vi "temp_dir_generate.vi"(8 "error in (no error)":errorcluster, 11 "temp_dir_config":T1) -> (0 "error out":errorcluster, 3 "temp_dir":path)   [LabVIEW 2015, in "lv-post-installer.lvlib"]
uses:
  lv-post-installer.lvlib
  _controls/temp_dir_config.ctl
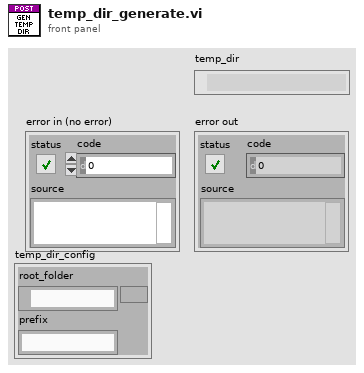
[diagram p1: front panel]
types:
  T1 = typedef "lv-post-installer.lvlib/temp_dir_config.ctl" = cluster{"root_folder":path, "prefix":string}
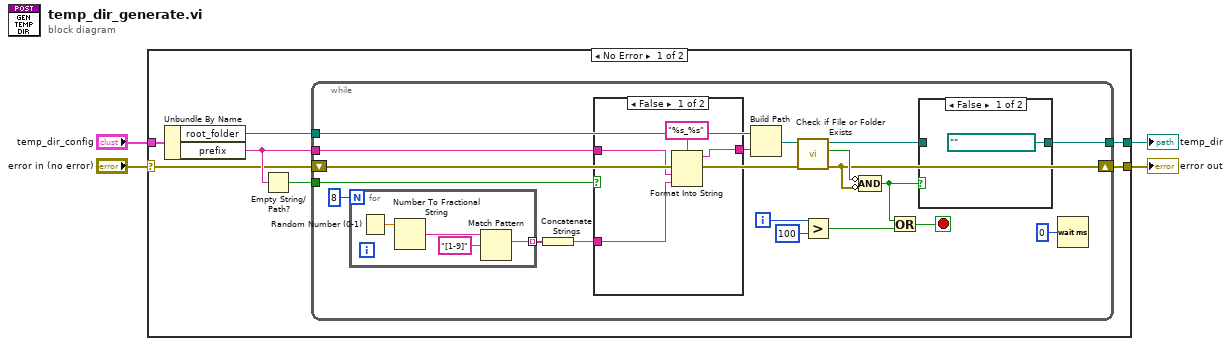
[diagram p0: block diagram]
diagram:
  n1 = case shown="No Error" "error in (no error)" {
    selector: "error in (no error)" -> [w5 w42]
    tunnel: [w8 _] -> w3
    tunnel: [w7 w42] -> w2
    tunnel: "temp_dir_config" -> [w6 _]
    frame No Error {
      n2 = Unbundle By Name(w6) -> ("root_folder"=w11:path, "prefix"=w10:string)
      n3 = Empty String/Path?(string/path=w10) -> (empty?=w9:bool)
      n4 = while {
        tunnel: w10 -> [w27]
        tunnel: w11 -> [w28]
        tunnel: w9 -> [w26]
        shift-right: [w21] -> w7
        shift-left: w5 -> [w12]
        tunnel: [w14] -> w8
        i -> [w19]
        stop <- w20 stop-if-true
        n5 = for {
          N: 8 -> [_]
          tunnel: [w31] -> w30 mode=indexing
          n6 = Random Number (0-1)() -> (number: 0 to 1=w34:dbl)
          n7 = Number To Fractional String(number=w34) -> (F-format string=w33:string)  [unwired: 3 in]
          n8 = Match Pattern(string=w33, regular expression="[1-9]") -> (match substring=w31:string)  [unwired: 1 in, 3 out]
        }
        n9 = Concatenate Strings(w30) -> (w25:string)
        n10 = case shown="False" w26 {
          tunnel: w27 -> [w39 _]
          tunnel: w25 -> [w38 w41]
          tunnel: [w37 w41] -> w24
          frame False {
            n11 = Format Into String(format string="%s_%s", w39, w38) -> (resulting string=w37:string)  [unwired: 2 in, 1 out]
          }
          frame True {
          }
        }
        n12 = Build Path(base path=w28, name or relative path=w24) -> (appended path=w23:path)
        n13 = call <vilib>:"Check if File or Folder Exists.vi"("error in (no error)"=w12, "path"=w23) -> ("error out"=w21:errorcluster, "file or folder exists?"=w22:bool, "dup path"=w15:path)  [unwired: 7 in]
        n14 = Greater?(x=w19, y=100) -> (0:w17:bool)
        n15 = Compound Arithmetic op=AND(invert w22, invert w21) -> (w16:bool)
        n16 = Or(x=w16, y=w17) -> (x .or. y?=w20:bool)
        n17 = case shown="False" w16 {
          tunnel: w15 -> [_ w36]
          tunnel: [path "" ("dup path") w36] -> w14
          frame False {
          }
          frame True {
          }
        }
        n18 = Wait (ms)(milliseconds to wait=u32 0) -> ()  [unwired: 1 out]
      }
    }
    frame Error {
    }
  }
  "error out" <- w2
  "temp_dir" <- w3
